vi "tb_interpolation_fft_transfer_compile.vi"() -> ()   [LabVIEW 2011]
uses:
  <vilib>/Platform/TimedLoop/XDataNode/XDataNode.xnode
  <vilib>/Platform/TimedLoop/XDataNode/nitl_modes.ctl
  <vilib>/Platform/TimedLoop/XDataNode/XDNodeRunTimeDep.lvlib
  <vilib>/Platform/TimedLoop/XDataNode/wakeup.ctl
  <vilib>/Platform/TimedLoop/XDataNode/timing_clust.ctl
  <vilib>/rvi/DataTransferAndStorage/Container/XNode/niFpgaContainer.xnode
  <vilib>/rvi/FXPMathLib/FxpInterpret/XNode/nifxpmath_Interpret.xnode
  <vilib>/eio/EIONode/EIONode.xnode
  <userlib>/FPGA Library/Code Development/Signal Processing/Interpolation Block/Controls/Interpolation Input Data.ctl
  <vilib>/rvi/FXPMathLib/basic elements/FxpDiscreteDelay/XNode/nifxpmath_DiscreteDelay.xnode
  <vilib>/rvi/FIFO/Fifo_Resource/nirvififoEmulationRead.vi
  <vilib>/rvi/FIFO/Fifo_Resource/nirvififoEmulationWrite.vi
  <vilib>/rvi/FIFO/Fifo_Resource/nirvififoEmulationGetNumberOfElementsToRead.vi
  <vilib>/rvi/interface/RandomDataEmulation/nirviRandomDataFpgaReadWriteTemplate.vi
  <vilib>/rvi/eio/common/nirviEmuTemplateMethod_errors.vi
  <userlib>/FPGA Library/Code Development/Signal Processing/FFT Block/FFT/Controls/FFT States.ctl
  <userlib>/FPGA Library/Code Development/Signal Processing/FFT Block/FFT/Controls/FFT Parameters.ctl
panel:
  in  "Trigger?":bool
  out "Time Out":bool
  out "Interp Loop Overflow":bool
  out "Current FFT State":T1
  out "FFT Status":T2
  in  "Address":u32
  in  "Data":T3 {"x[n].ResampleInfo"."Lambda" format="%.18g"; "x[n-1].ResampleInfo"."Lambda" format="%.18g"}
  in  "Write?":bool
  in  "FFT Parameters":T4={"Direction"=TRUE, "scale_sch"=85.0, "Flush Length"=0} {"scale_sch" format="%.0b"}
  in  "FFT State":cluster{"FFT State":T1, "Set FFT State?":bool}
  out "acq timed out?":bool
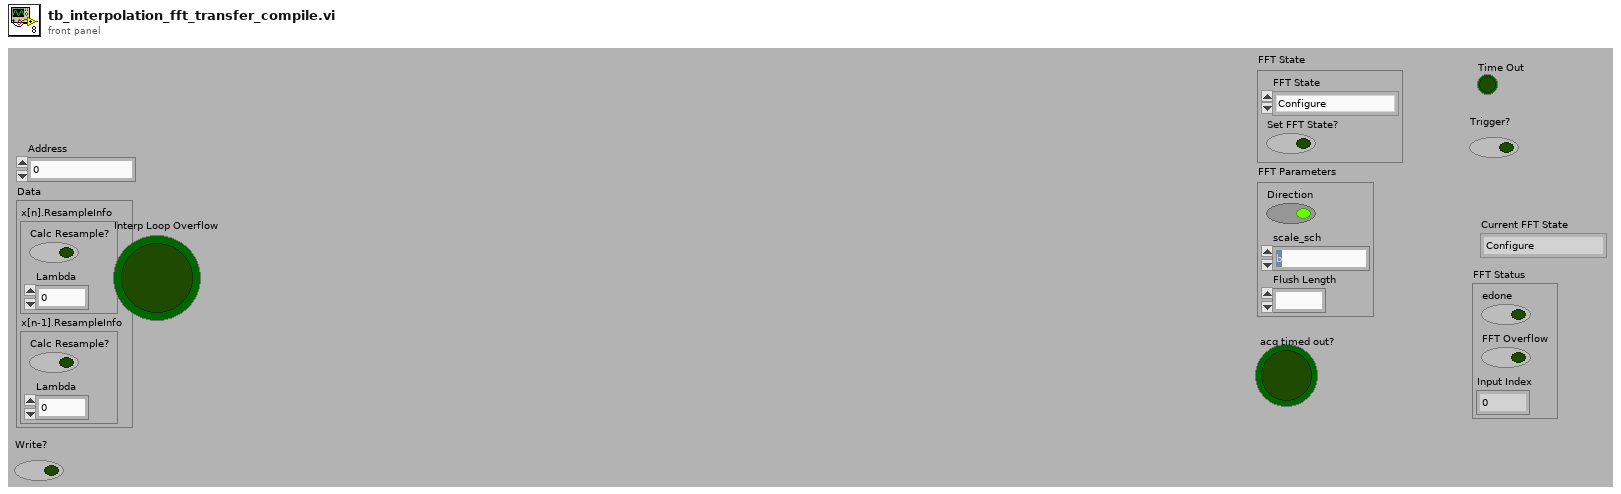
[diagram p1: front panel]
types:
  T1 = typedef "FFT States.ctl" = enum8{"Configure", "Start FFT processing", "Process", "Unload Last FFT", "Reset"}
  T2 = cluster{"edone":bool, "FFT Overflow":bool, "Input Index":fxp<+,9,9>}
  T3 = cluster{"x[n].ResampleInfo":cluster{"Calc Resample?":bool, "Lambda":fxp<+/-,18,1>}, "x[n-1].ResampleInfo":cluster{"Calc Resample?":bool, "Lambda":fxp<+/-,18,1>}}
  T4 = typedef "FFT Parameters.ctl" = cluster{"Direction":bool, "scale_sch":fxp<+,10,10>, "Flush Length":u16}
  T5 = typedef "XDNodeRunTimeDep.lvlib/timing_clust.ctl" = cluster{"Expected End [f-1]":u64, "Actual End [f-1]":u64, "Finished Late? [f-1]":bool, "Expected End [i-1]":u64, "Actual End [i-1]":u64, "Finished Late? [i-1]":bool, "Expected Start [i]":u64, "Actual Start [i]":u64, "Expected Start [f]":u64, "Actual Start [f]":u64, "Source Name":string, "Structure Name":string, "Period":i64, "Deadline":i64, "Offset":i64, "Start":i64, "Priority":i32, "Timeout":i32, "Mode":T6, "Wakeup Reason":T7, "Error":errorcluster, "Source Type":string, "Secondary Source Type":string, "Global End Time":u64, "Global Start Time":u64, "Frame Duration":u64, "Iteration Duration":u64, "Assigned CPU":i32, "I/O Scan Engine Mode":u32}
  T6 = typedef "XDNodeRunTimeDep.lvlib/nitl_modes.ctl" = enum32{"No Change", "Process missed periods, maintain original phase", "Discard missed periods, maintain original phase", "Process missed periods, ignore original phase", "Discard missed periods, ignore original phase"}
  T7 = typedef "XDNodeRunTimeDep.lvlib/wakeup.ctl" = enum32{"Normal", "Aborted", "Asynchronous wakeup", "Timing source error", "Timed loop error", "Timeout"}
  T8 = typedef "Interpolation Input Data.ctl" = fxp<+/-,18,1>
  T9 = typedef "Interpolation Output Data.ctl" = fxp<+/-,19,1>
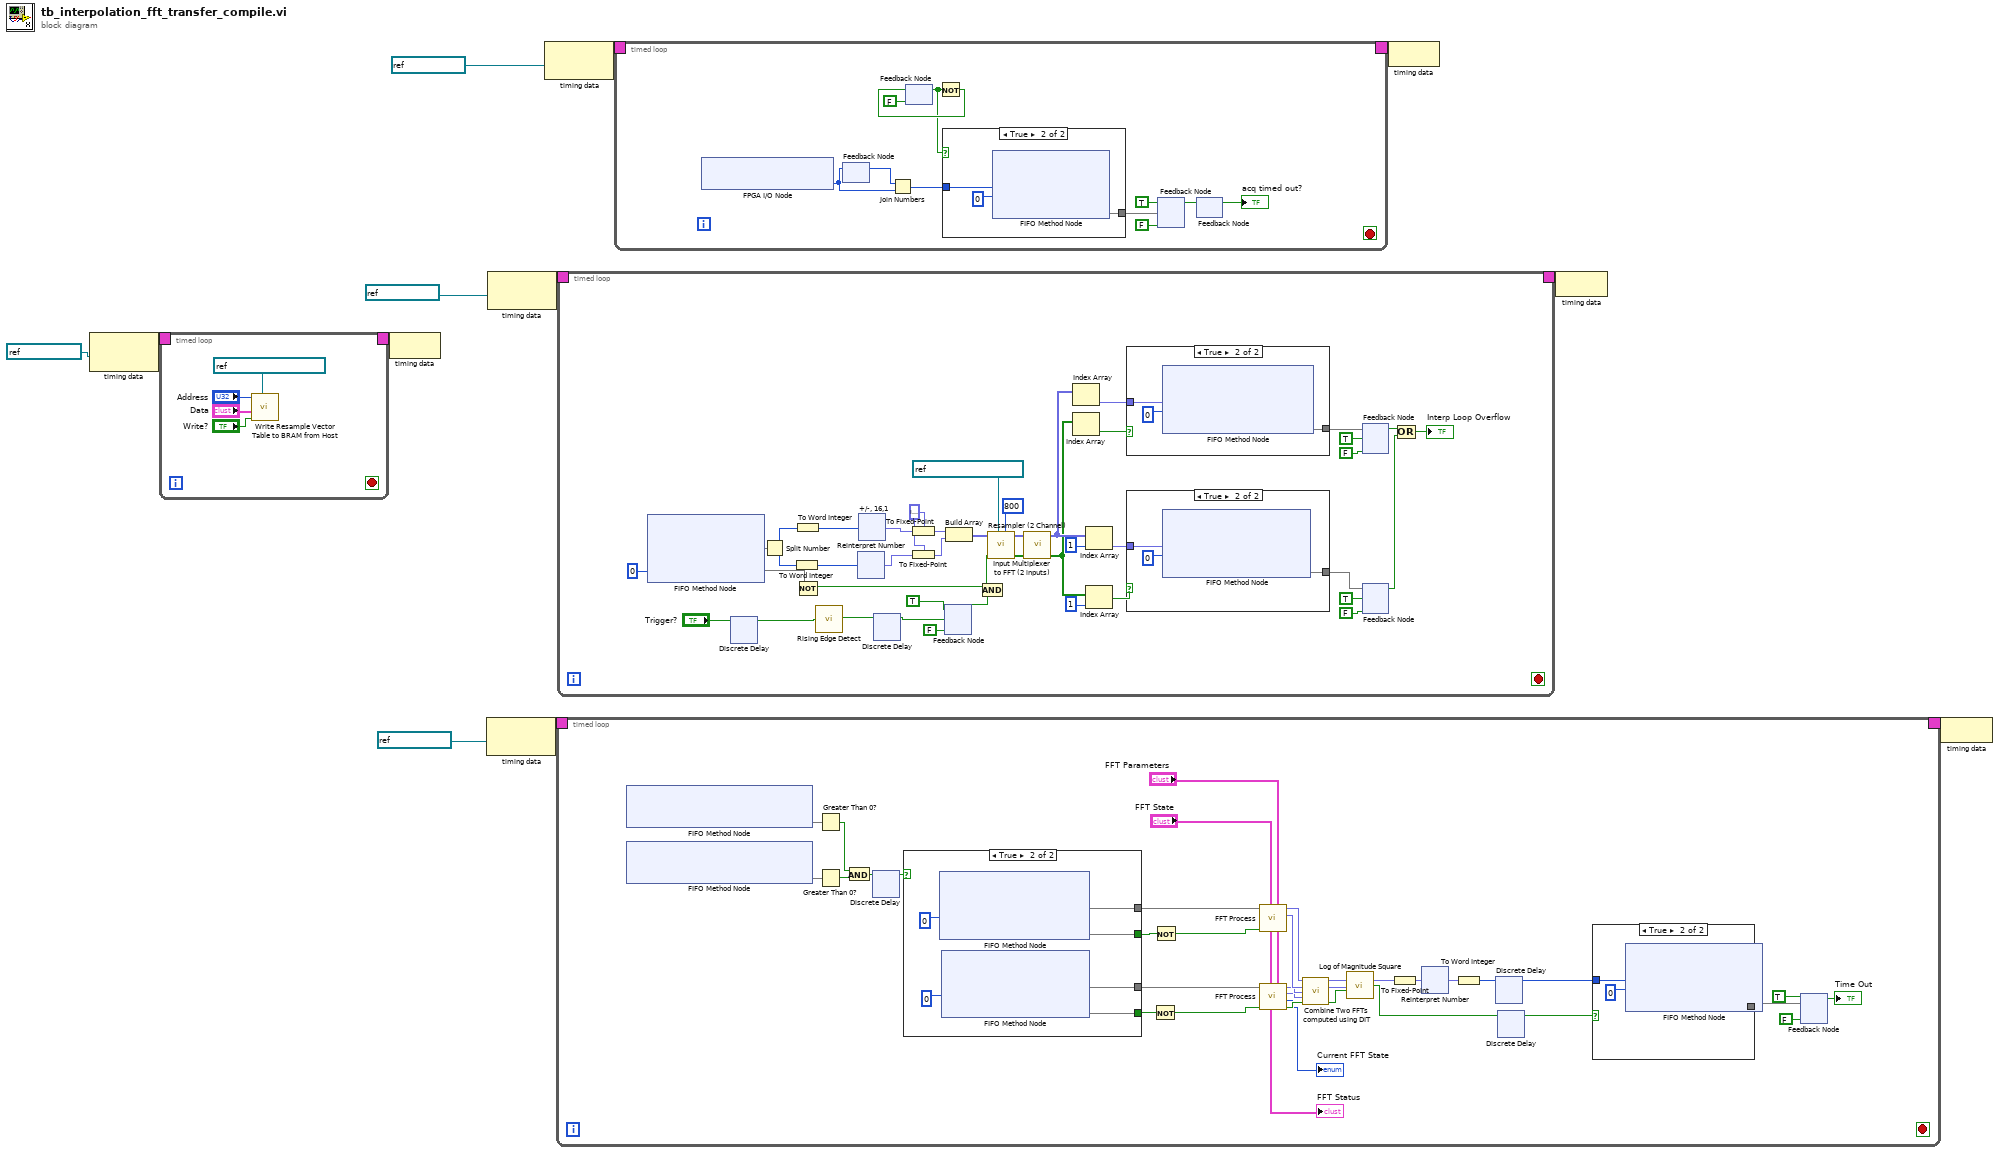
[diagram p0: block diagram]
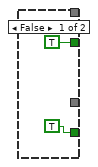
[diagram p6: hidden frame]
diagram:
  n1 = node-c288(refnum<k21> "126.67MHz" ("Source Name")) -> (w6:T5)
  n2 = timed-loop {
    timing: w6 -> [_]
    timing-out: [_] -> w5
    stop <- _ stop-if-true
    n3 = call <userlib>:"Write Resample Vector Table to BRAM from Host.vi"("Resample Table"=refnum<k21> "Interpolation Table", "Write?"="Write?", "Data"="Data", "Address"="Address") -> ()  [unwired: 8 in]
  }
  n4 = node-c288(w5) -> ()
  n5 = node-c288(refnum<k21> "126.67MHz" ("Source Name")) -> (w12:T5)
  n6 = node-c288(refnum<k21> "126.67MHz" ("Source Name")) -> (w3:T5)
  n7 = node-c288(refnum<k21> "ADC Clock" ("Source Name")) -> (w10:T5)
  n8 = timed-loop {
    timing: w12 -> [_]
    timing-out: [_] -> w11
    stop <- _ stop-if-true
    n9 = xnode ("FIFO Method Node")() -> ("Number of Elements to Read"=w49)  [unwired: 1 in, 1 out]
    n10 = xnode ("FIFO Method Node")() -> ("Number of Elements to Read"=w48)  [unwired: 1 in, 1 out]
    n11 = Greater Than 0?(x=w49) -> (x > 0?=w47:bool)
    n12 = Greater Than 0?(x=w48) -> (x > 0?=w46:bool)
    n13 = And(x=w47, y=w46) -> (x .and. y?=w45:bool)
    n14 = xnode "Discrete Delay"("D"=w45) -> ("Q"=w23:bool)
    n15 = case shown="True" w23 {
      tunnel: [TRUE ("Timed Out?") w62] -> w53
      tunnel: [_ w61] -> w28
      tunnel: [_ w60] -> w27
      tunnel: [TRUE ("Timed Out?") w59] -> w52
      frame False {
      }
      frame True {
        n16 = xnode ("FIFO Method Node")("Timeout"=0) -> ("Element"=w61, "Timed Out?"=w62)  [unwired: 1 in, 1 out]
        n17 = xnode ("FIFO Method Node")("Timeout"=0) -> ("Element"=w60, "Timed Out?"=w59)  [unwired: 1 in, 1 out]
      }
    }
    n18 = Not(x=w52) -> (.not. x?=w29:bool)
    n19 = Not(x=w53) -> (.not. x?=w50:bool)
    n20 = call <userlib>:"FFT Process.vi"("FFT Parameters"="FFT Parameters", "FFT State"="FFT State", "Input Valid"=w50, "Real Data In"=w28) -> ("Imag Data Out"=w41:fxp<+/-,16,1>, "Real Data Out"=w42:fxp<+/-,16,1>)  [unwired: 2 in, 4 out]
    n21 = call <userlib>:"FFT Process.vi"("FFT Parameters"="FFT Parameters", "FFT State"="FFT State", "Input Valid"=w29, "Real Data In"=w27) -> ("Output Valid"=w35:bool, "Current FFT State"=→"Current FFT State":T1, "Imag Data Out"=w39:fxp<+/-,16,1>, "Real Data Out"=w40:fxp<+/-,16,1>, "FFT Status"=→"FFT Status":T2)  [unwired: 2 in, 1 out]
    n22 = call <userlib>:"Combine Two FFTs computed using DIT.vi"("Real FFT 1"=w42, "Imag FFT 1"=w41, "Real FFT 2"=w40, "Imag FFT 2"=w39, "Input Data Valid"=w35) -> ("Real FFT k"=w32:fxp<+/-,24,3>, "Imag FFT k"=w31:fxp<+/-,24,3>, "Output Valid"=w30:bool)  [unwired: 6 in, 2 out]
    n23 = call <userlib>:"Log of Magnitude Square.vi"("Real"=w32, "Imaginary"=w31, "Input Valid"=w30) -> ("Log Magnitude"=w25:fxp<+/-,34,12>, "Output Valid"=w43:bool)  [unwired: 11 in]
    n24 = To Fixed-Point(number=w25) -> (fixed-point=w33:fxp<+/-,16,8>)  [unwired: 1 in]
    n25 = xnode "Reinterpret Number"("x"=w33) -> ("y"=w51:fxp<+/-,16,16>)
    n26 = To Word Integer(number=w51) -> (16bit integer=w44:i16)
    n27 = xnode "Discrete Delay"("D"=w44) -> ("Q"=w24:i16)
    n28 = xnode "Discrete Delay"("D"=w43) -> ("Q"=w26:bool)
    n29 = case shown="True" w26 {
      tunnel: w24 -> [_ w56]
      tunnel: [_ w54] -> w22
      frame False {
      }
      frame True {
        n30 = xnode ("FIFO Method Node")("Element"=w56, "Timeout"=0) -> ("Timed Out?"=w54)  [unwired: 1 in, 1 out]
      }
    }
    n31 = feedback-in #1(TRUE, w22) -> ()
    n32 = feedback #1(FALSE) -> (→"Time Out":bool)
  }
  n33 = timed-loop {
    timing: w3 -> [_]
    timing-out: [_] -> w2
    stop <- _ stop-if-true
    w92 = T8 0.0 ("Interpolate.Input Data")
    n34 = xnode ("FIFO Method Node")("Timeout"=0) -> ("Element"=w95, "Timed Out?"=w90)  [unwired: 1 in, 1 out]
    n35 = xnode "Discrete Delay"("D"="Trigger?") -> ("Q"=w79:bool)
    n36 = Split Number(x=w95) -> (hi(x)=w84:u16, lo(x)=w83:u16)
    n37 = To Word Integer(number=w83) -> (16bit integer=w81:i16)
    n38 = To Word Integer(number=w84) -> (16bit integer=w82:i16)
    n39 = Not(x=w90) -> (.not. x?=w73:bool)
    n40 = call <userlib>:"Rising Edge Detect.vi"("signal"=w79) -> ("edge detected"=w78:bool)  [unwired: 14 in]
    n41 = xnode "Reinterpret Number"("x"=w81) -> ("y"=w88:fxp<+/-,16,1>)
    n42 = xnode "+/-, 16,1"("x"=w82) -> ("y"=w86:fxp<+/-,16,1>)
    n43 = xnode "Discrete Delay"("D"=w78) -> ("Q"=w77:bool)
    n44 = To Fixed-Point(fixed-point type=w92, number=w86) -> (fixed-point=w87:T8)
    n45 = To Fixed-Point(fixed-point type=w92, number=w88) -> (fixed-point=w93:T8)
    n46 = feedback-in #2(TRUE, w77) -> ()
    n47 = feedback #2(FALSE) -> (w74:bool)
    n48 = Build Array(w87, w93) -> (w91:T8[])
    n49 = And(x=w73, y=w74) -> (x .and. y?=w72:bool)
    n50 = call <userlib>:"Resampler (2 Channel).vi"("CalibrationTable Length-1"=u16 800, "ResampleVectorInfo"=refnum<k21> "Interpolation Table", "DataValid"=w72, "Input Data"=w91) -> ("Data Valid"=w113:bool[], "Interpolated Data"=w114:T9[])  [unwired: 6 in]
    n51 = call <userlib>:"Input Multiplexer to FFT (2 inputs).vi"("Input Data Valid Array"=w113, "Input Data"=w114) -> ("Output Data Valid Array"=w108:bool[], "Interchanged Data"=w110:T9[])  [unwired: 8 in]
    n52 = Index Array(array=w110) -> (element=w112:T9)  [unwired: 1 in]
    n53 = Index Array(array=w108) -> (element=w111:bool)  [unwired: 1 in]
    n54 = Index Array(array=w110, index=1) -> (element=w109:T9)
    n55 = Index Array(array=w108, index=1) -> (element=w107:bool)
    n56 = case shown="True" w111 {
      tunnel: w112 -> [_ w124]
      tunnel: [_ w122] -> w104
      frame False {
      }
      frame True {
        n57 = xnode ("FIFO Method Node")("Element"=w124, "Timeout"=0) -> ("Timed Out?"=w122)  [unwired: 1 in, 1 out]
      }
    }
    n58 = case shown="True" w107 {
      tunnel: w109 -> [_ w121]
      tunnel: [_ w119] -> w101
      frame False {
      }
      frame True {
        n59 = xnode ("FIFO Method Node")("Element"=w121, "Timeout"=0) -> ("Timed Out?"=w119)  [unwired: 1 in, 1 out]
      }
    }
    n60 = feedback-in #3(w104, TRUE) -> ()
    n61 = feedback #3(FALSE ("Timed Out?")) -> (w100:bool)
    n62 = feedback #4(FALSE ("Timed Out?")) -> (w97:bool)
    n63 = feedback-in #4(w101, TRUE) -> ()
    n64 = Or(x=w100, y=w97) -> (x .or. y?=→"Interp Loop Overflow":bool)
  }
  n65 = timed-loop {
    timing: w10 -> [_]
    timing-out: [_] -> w9
    stop <- _ stop-if-true
    n66 = xnode "FPGA I/O Node"() -> ("IO Module\\AI 0 Data"=w128:i16)  [unwired: 1 in, 1 out]
    n67 = feedback-in #5(w128) -> ()
    n68 = feedback #5() -> (w129:i16)  [unwired: 1 in]
    n69 = Join Numbers(hi=w129, lo=w128) -> ((hi.lo)=w130:u32)
    n70 = feedback #6(FALSE) -> (w131:bool)
    n71 = Not(x=w131) -> (.not. x?=w137:bool)
    n72 = feedback-in #6(w137) -> ()
    n73 = case shown="True" w131 {
      tunnel: w130 -> [_ w140]
      tunnel: [_ w138] -> w134
      frame False {
      }
      frame True {
        n74 = xnode ("FIFO Method Node")("Element"=w140, "Timeout"=0) -> ("Timed Out?"=w138)  [unwired: 1 in, 1 out]
      }
    }
    n75 = feedback-in #7(TRUE, w134) -> ()
    n76 = feedback #7(FALSE) -> (w132:bool)
    n77 = feedback-in #8(w132) -> ()
    n78 = feedback #8() -> (→"acq timed out?":bool)  [unwired: 1 in]
  }
  n79 = node-c288(w9) -> ()
  n80 = node-c288(w2) -> ()
  n81 = node-c288(w11) -> ()
